vi "Write Sample Container.vi"(8 "error in (no error)":errorcluster, 10 "Sample Container":T1, 11 "Capillary Line in":refnum<class "Capillary Line.lvclass">) -> (0 "error out":errorcluster, 3 "Capillary Line out":refnum<class "Capillary Line.lvclass">)   [LabVIEW 2015, in "cRIO-Carbondioxide.lvlib" / "CO2-Actor.lvlib" / "Capillary Line.lvclass"]
uses:
  Capillary Line.lvclass
  Controls/Sample Container.ctl
  subs/Sample/Sample.lvclass
  Capillary Line.lvclass/Capillary Line.ctl
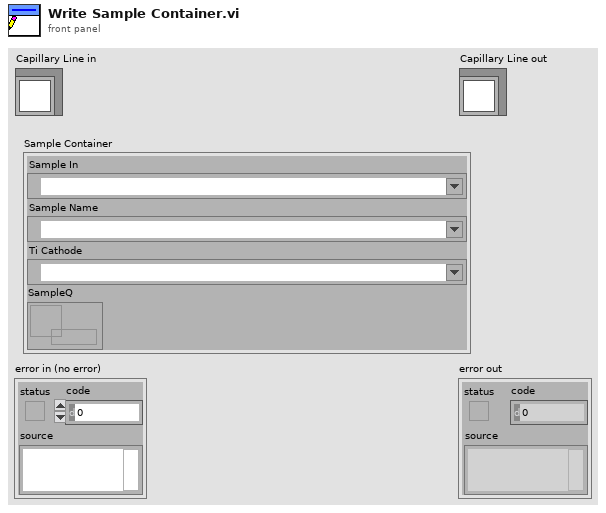
[diagram p1: front panel]
types:
  T1 = typedef "Sample Container.ctl" = cluster{"Sample In":refnum<k21>, "Sample Name":refnum<k21>, "Ti Cathode":refnum<k21>, "SampleQ":refnum<queue>}
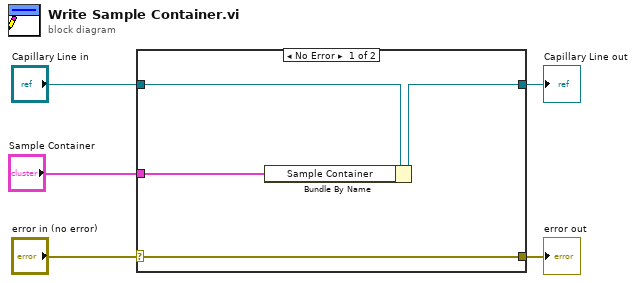
[diagram p0: block diagram]
diagram:
  n1 = case shown="No Error" "error in (no error)" {
    selector: "error in (no error)" -> [w9 w10]
    tunnel: [w9 w10] -> w4
    tunnel: [w7 w11] -> w2
    tunnel: "Capillary Line in" -> [w8 w11]
    tunnel: "Sample Container" -> [w6 _]
    frame No Error {
      n2 = Bundle By Name(cluster=w8, "Sample Container"=w6) -> (w7:refnum<class "Capillary Line.lvclass">)
    }
    frame Error {
    }
  }
  "error out" <- w4
  "Capillary Line out" <- w2
